vi "2sComplement.vi"   [LabVIEW 2012]
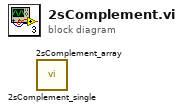
[diagram p0: block diagram]
diagram:
  n1 = call "2sComplement_single.vi"() -> ()  [unwired: 2 in, 1 out]
  n2 = call "2sComplement_array.vi"() -> ()  [unwired: 2 in, 1 out]
